vi "audio-stim2.vi"(11 "Stimulus List":dbl[][](array[numeric])) -> (3 "Playing":bool caption="Playing stimulus")   [LabVIEW 2009]
uses:
  <vilib>/DAQmx/create/channels.llb/DAQmx Create Channel (DO-Digital Output).vi
  <vilib>/DAQmx/write.llb/DAQmx Write (Digital U16 1Chan 1Samp).vi
  <vilib>/DAQmx/create/channels.llb/DAQmx Create Channel (AO-Voltage-Basic).vi
  <vilib>/DAQmx/write.llb/DAQmx Write (Analog Wfm 1Chan NSamp).vi
  <vilib>/DAQmx/configure/timing.llb/DAQmx Timing (Use Waveform).vi
panel:
  in  "Total Trials":i32 min=1 step=1
  out "Total Played":i32 caption="Total Played or Cued"
  in  "Save Stimulus List":bool
  in  "Load Stimulus List":bool
  out "Stimulus List Path":path
  out "Log File Path":path
  in  "Play Interval Jitter (s)":dbl
  in  "Play Interval (s)":dbl
  out "error out":errorcluster
  in  "DO Ports":tag caption="DO Ports\n(\"browse\" and select two 8 bit ports)"
  in  "Sound AO Channel":tag
  out "Curr Param":dbl[](array[numeric]) caption="Current (or Cued) Trial Parameters"
  in  "Sampling Rate":dbl
  in  "stop":bool
  in  "Play":bool
  out "Current (or Cued) Waveform":waveform(dbl)(graph)
  out "Waiting":bool
  # "Stim#, Stim Type, Duration, Amplitude, Param 1, Param 2, Param 3, Param 4"
  # "Stim Type 1 DC (no parameters, just amplitude)"
  # "Stim Type 3 Pure Tone (param1 = frequency)"
  # "Stim Type 4 FM Sweep (param1 = start frequency, param2 = end frequency)"
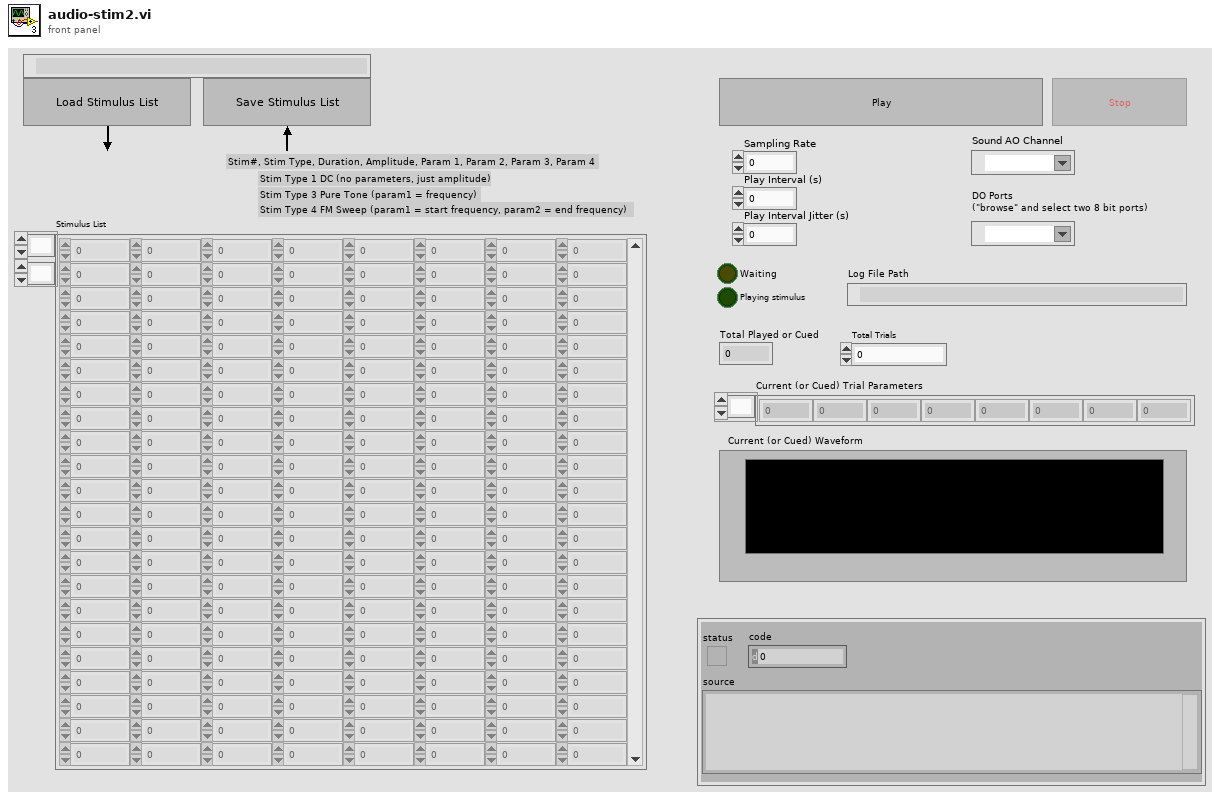
[diagram p1: front panel]
types:
  T1 = enum8{"Enabled", "Disabled", "Disabled and Grayed Out"}
  T2 = cluster{"Sampling Rate":dbl, "Value 3":dbl, dbl, "Value 2":dbl}
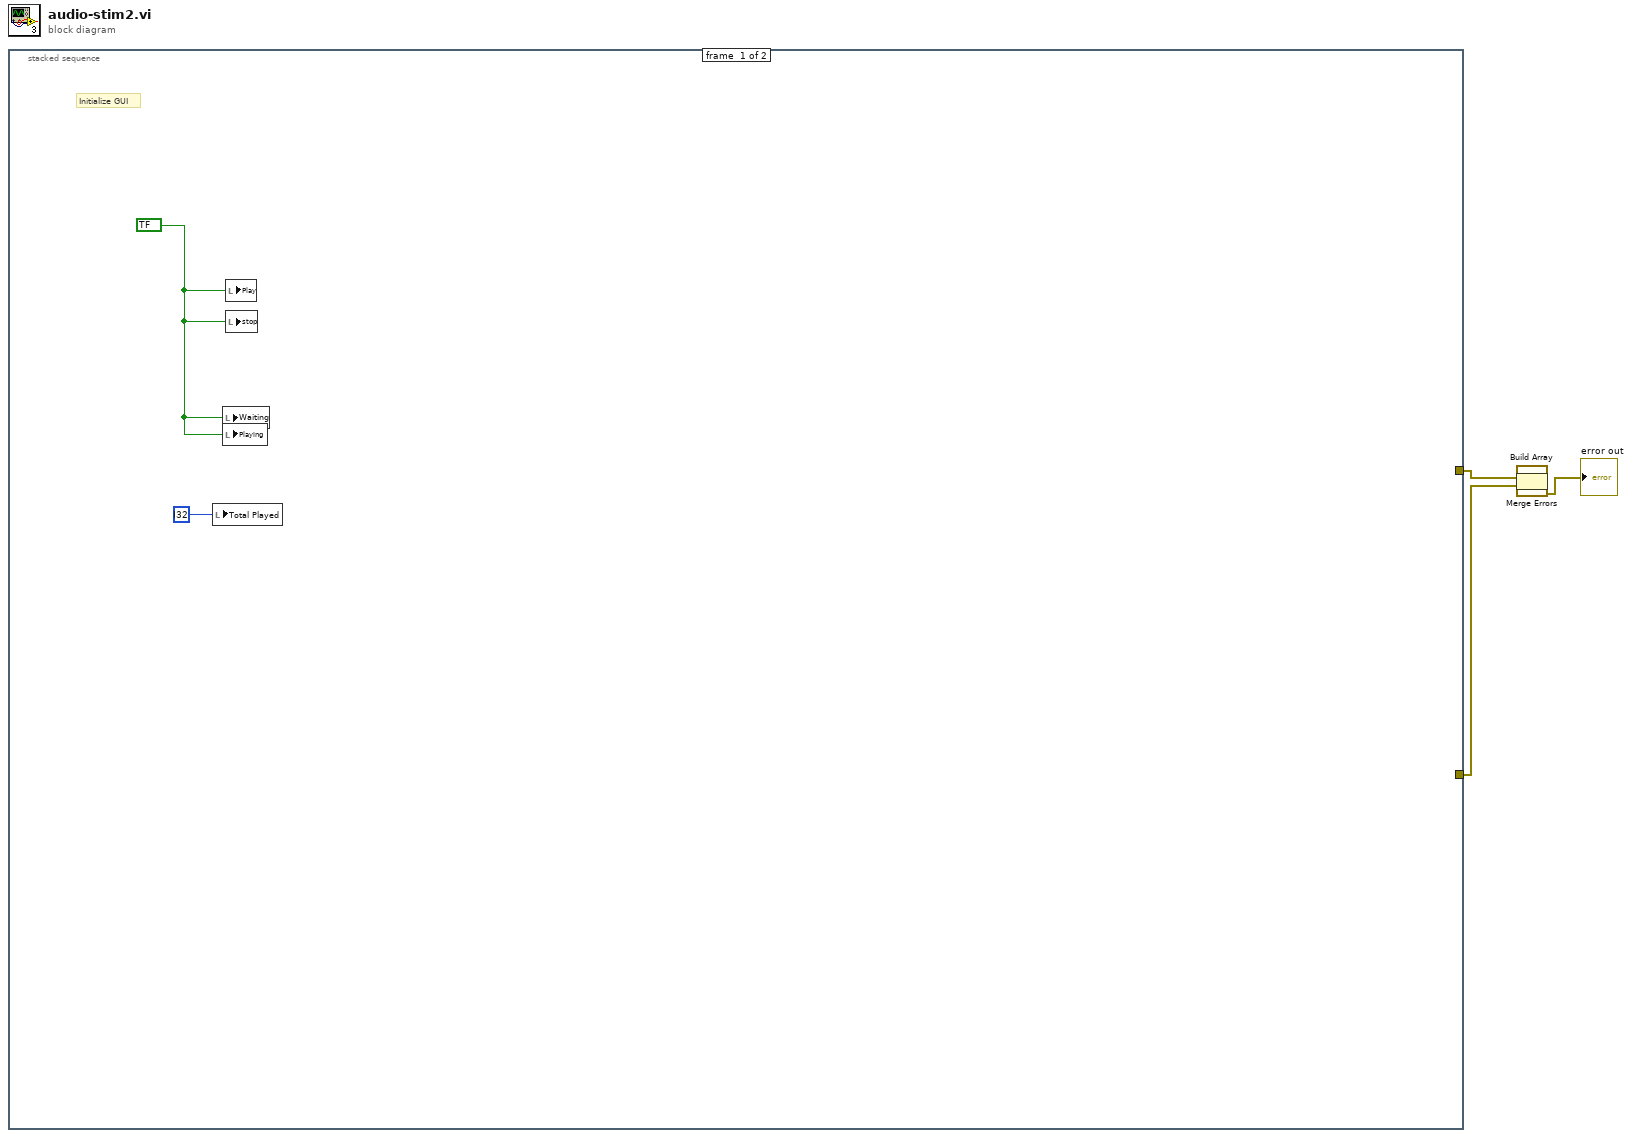
[diagram p0: block diagram]
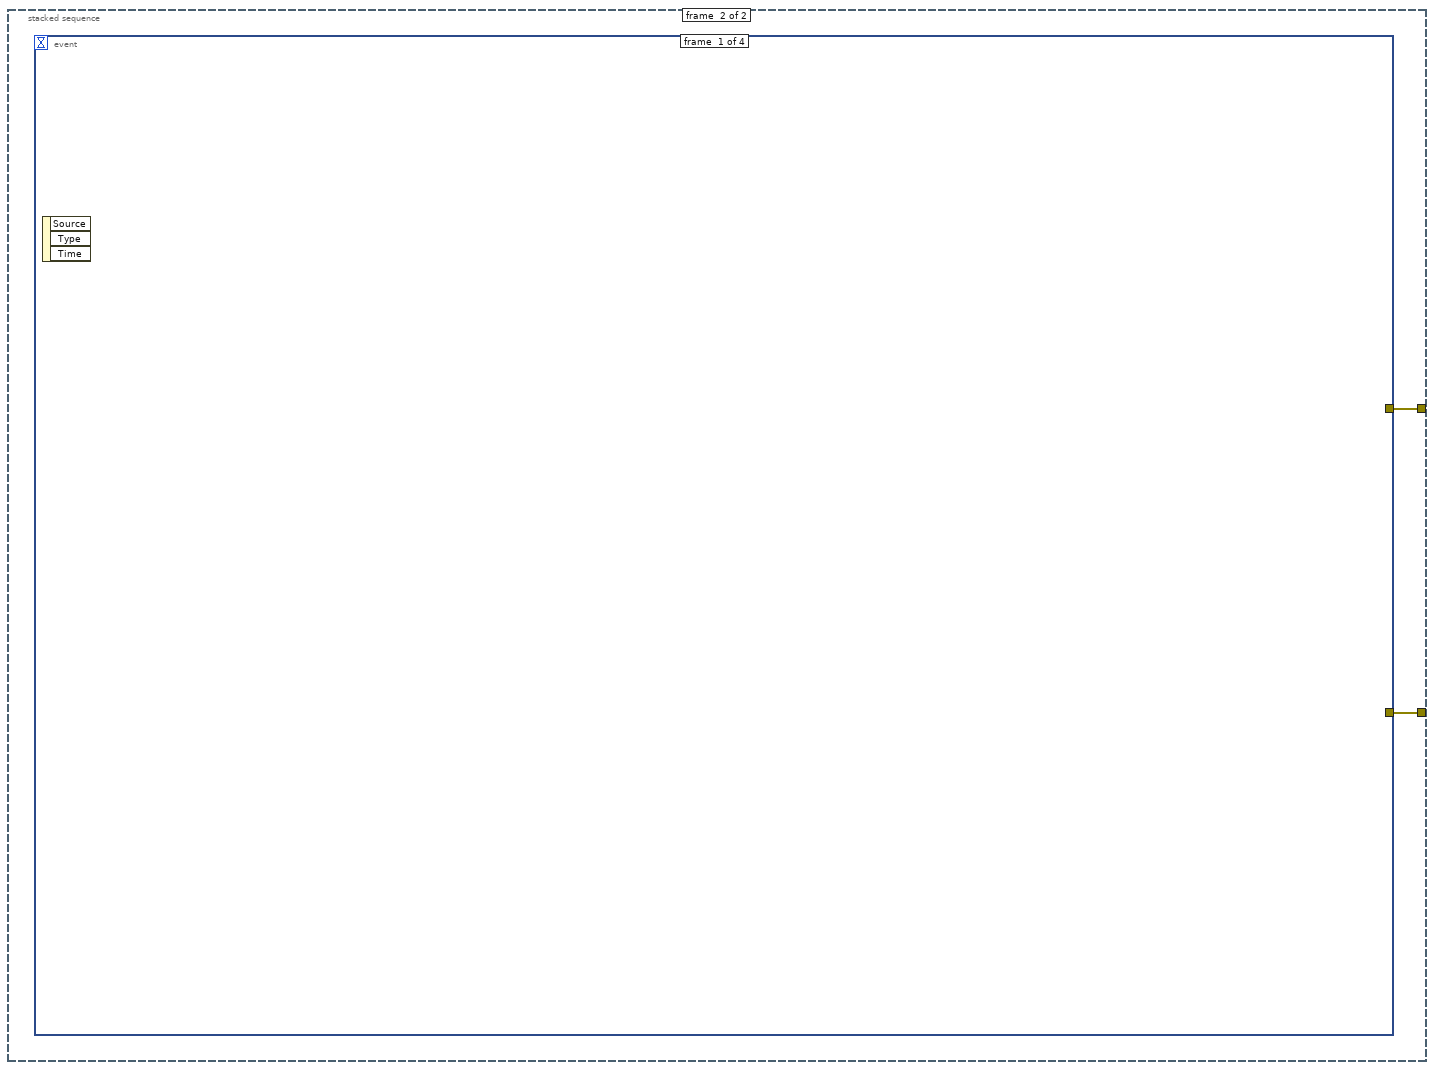
[diagram p2: hidden frame]
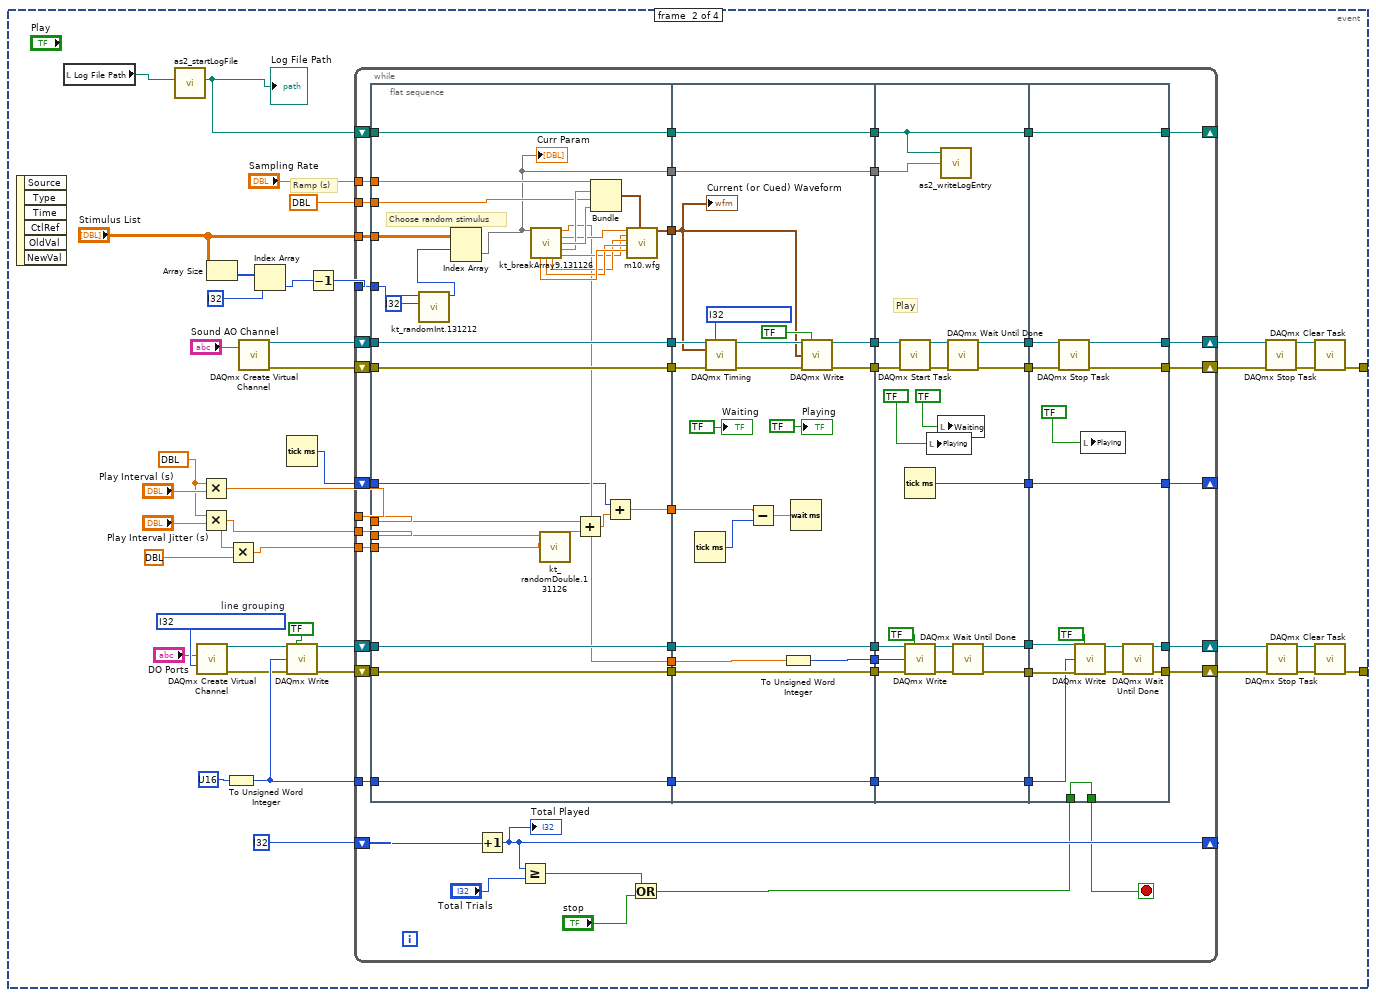
[diagram p3: hidden frame]
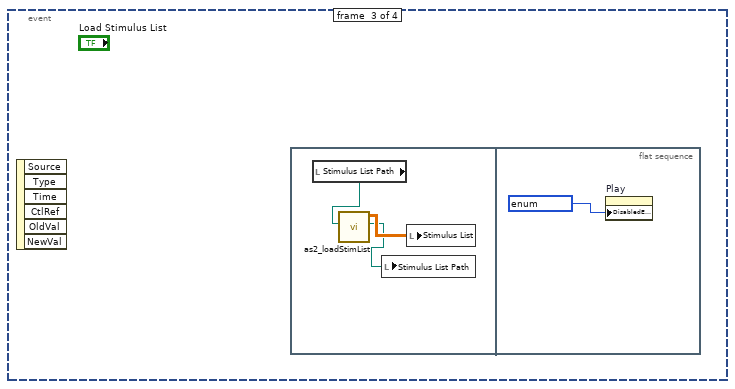
[diagram p4: hidden frame]
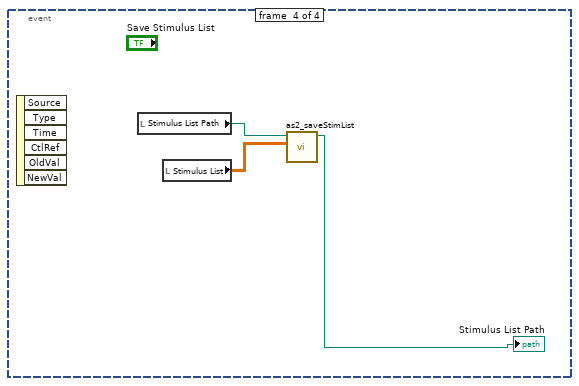
[diagram p5: hidden frame]
diagram:
  n1 = stacked-sequence {
    tunnel: [_ w8] -> w4
    tunnel: [_ w7] -> w3
    frame #0 {
      w6 = bool ? ("Play")
      # "Initialize GUI"
      n2 = local write "Total Played"(i32 ? ("Total Played")) -> ()
      n3 = local write "Waiting"(w6) -> ()
      n4 = local write "Playing"(w6) -> ()
      n5 = local write "Play"(w6) -> ()
      n6 = local write "stop"(w6) -> ()
    }
    frame #1 {
      n7 = event shown="[1] \"Play\": Value Change" {
        selector: _ -> [_ _ _ _]
        dyn-events: _ -> [_ _ _ _]
        timeout: _ -> [_ _ _ _]
        tunnel: [_ w25 _ _] -> w8
        tunnel: [_ w24 _ _] -> w7
        event #0 {
          n8 = event-data() -> ()  [unwired: 1 in, 3 out]
        }
        event #1 {
          w18 = dbl ? ("y")
          w45 = i32 ? items=["one channel for each line", "one channel for all lines"]  # line grouping
          # "Ramp (s)"
          n9 = event-data() -> ()  [unwired: 1 in, 6 out]
          n10 = local read "Log File Path"() -> (w13:path)
          n11 = call "as2_startLogFile.vi"("Path In"=w13) -> ("Path"=w12:path)  [unwired: 5 in, 1 out]
          "Log File Path" <- w12
          n12 = call-poly <vilib>:"DAQmx Create Virtual Channel.vi"("lines"="DO Ports", "line grouping"=w45) -> ("task out"=w23:refnum<k21>, "error out"=w22:errorcluster)  [unwired: 12 in]
          n13 = Multiply(x=w18, y="Play Interval (s)") -> (x*y=w17:dbl)
          n14 = Multiply(x=w18, y="Play Interval Jitter (s)") -> (x*y=w15:dbl)
          n15 = Array Size(array="Stimulus List") -> (size(s)=w43:i32[])
          n16 = To Unsigned Word Integer(number=u16 ? ("data")) -> (unsigned 16bit integer=w28:u16)
          n17 = Multiply(x=w15, y=dbl ?) -> (x*y=w16:dbl)
          n18 = call-poly <vilib>:"DAQmx Create Virtual Channel.vi"("physical channels"="Sound AO Channel") -> ("task out"=w27:refnum<k21>, "error out"=w26:errorcluster)  [unwired: 13 in]
          n19 = Index Array(array=w43, index=i32 ?) -> (element=w11:i32)
          n20 = Tick Count (ms)() -> (millisecond timer value=w14:u32)
          n21 = call-poly <vilib>:"DAQmx Write.vi"("task/channels in"=w23, "auto start"=bool ?, "data"=w28, "error in"=w22) -> ("task out"=w32:refnum<k21>, "error out"=w31:errorcluster)  [unwired: 9 in, 1 out]
          n22 = Decrement(x=w11) -> (x-1=w10:i32)
          n23 = while {
            tunnel: "Stimulus List" -> [w73]
            tunnel: "Sampling Rate" -> [w72]
            tunnel: dbl ? -> [w71]
            shift-right: [w98] -> w37
            shift-left: w27 -> [w96]
            shift-right: [w97] -> w36
            shift-left: w26 -> [w95]
            shift-right: [w87] -> w41
            shift-left: w32 -> [w94]
            shift-right: [w86] -> w40
            shift-left: w31 -> [w81]
            shift-right: [w52] -> _
            shift-left: i32 ? ("data") -> [w53]
            tunnel: w28 -> [w84]
            shift-right: [w68] -> _
            shift-left: w14 -> [w67]
            tunnel: w17 -> [w63]
            tunnel: w16 -> [w64]
            tunnel: w15 -> [w65]
            shift-right: [w56] -> _
            shift-left: w12 -> [w62]
            tunnel: w10 -> [w55]
            stop <- w50 stop-if-true
            n24 = flat-sequence {
              tunnel: [w130] -> w79
              tunnel: [w129] -> w78
              tunnel: [w128] -> w77
              tunnel: [w127] -> w76
              tunnel: [w126] -> w75
              tunnel: [w118] -> w74
              tunnel: [w115] -> w70
              tunnel: [w112] -> w66
              tunnel: [w106] -> w61
              tunnel: [w105] -> w60
              tunnel: w55 -> [w104]
              tunnel: w62 -> [w106]
              tunnel: w63 -> [w107]
              tunnel: w64 -> [w110]
              tunnel: w65 -> [w111]
              tunnel: w67 -> [w113]
              tunnel: w71 -> [w116]
              tunnel: w72 -> [w117]
              tunnel: w73 -> [w102]
              tunnel: w81 -> [w126]
              tunnel: w84 -> [w127]
              tunnel: w94 -> [w128]
              tunnel: w95 -> [w129]
              tunnel: w96 -> [w130]
              tunnel: [w141] -> w100
              tunnel: [w140] -> w99
              tunnel: [w150] -> w93
              tunnel: [w149] -> w88
              tunnel: [w148] -> w85
              tunnel: [w138] -> w80
              tunnel: w79 -> [w147]
              tunnel: w78 -> [w146]
              tunnel: w77 -> [w150]
              tunnel: w76 -> [w148]
              tunnel: w75 -> [w138]
              tunnel: w74 -> [w137]
              tunnel: w70 -> [w136]
              tunnel: w66 -> [w133]
              tunnel: w61 -> [w131]
              tunnel: w60 -> [w132]
              tunnel: [w132] -> w59
              tunnel: [w131] -> w58
              tunnel: w100 -> [w161]
              tunnel: w99 -> [w160]
              tunnel: w93 -> [w169]
              tunnel: [w163] -> w92
              tunnel: [w162] -> w91
              tunnel: [w166] -> w90
              tunnel: [w165] -> w89
              tunnel: w88 -> [w170]
              tunnel: w85 -> [w164]
              tunnel: [w164] -> w83
              tunnel: w80 -> [w155]
              tunnel: [w154] -> w69
              tunnel: w59 -> [w153]
              tunnel: w58 -> [w152]
              tunnel: [w152] -> w57
              tunnel: [w175] -> w97
              tunnel: [w176] -> w98
              tunnel: w92 -> [w178]
              tunnel: w91 -> [w177]
              tunnel: w90 -> [w186]
              tunnel: w89 -> [w185]
              tunnel: [w181] -> w87
              tunnel: [w180] -> w86
              tunnel: w83 -> [w179]
              tunnel: w69 -> [w174]
              tunnel: [w174] -> w68
              tunnel: w57 -> [w173]
              tunnel: [w173] -> w56
              tunnel: w51 -> [w172]
              tunnel: [w172] -> w50
              frame #0 {
                # "Choose random stimulus"
                n25 = call "kt_randomInt.131212.vi"("Min"=i32 ?, "Max"=w104) -> ("Random"=w101:i32)  [unwired: 9 in]
                n26 = Index Array(array=w102, index (row)=w101) -> (element=w105:dbl[])  [unwired: 1 in]
                "Curr Param" <- w105
                n27 = call "kt_breakArray9.131126.vi"("Current (or Cued Trial Parameters)"=w105) -> ("Value 0"=w115:dbl, "Value 1"=w119:dbl, "Value 2"=w121:dbl, "Value 3"=w120:dbl, "Value 7"=w125:dbl, "Value 6"=w124:dbl, "Value 5"=w123:dbl, "Value 4"=w122:dbl)  [unwired: 6 in, 1 out]
                n28 = call "kt_randomDouble.131126.vi"("Min"=w110, "Max"=w111) -> ("Random"=w108:dbl)  [unwired: 9 in]
                n29 = Add(x=w107, y=w108) -> (x+y=w109:dbl)
                n30 = Bundle("Sampling Rate"=w117, "Value 3"=w120, w116, "Value 2"=w121) -> (w114:T2)  [unwired: 1 in]
                n31 = Add(x=w113, y=w109) -> (x+y=w112:dbl)
                n32 = call "m10.wfg.vi"("Stimulus Type"=w119, "Param 0"=w122, "Param 1"=w123, "Param 2"=w124, "Param 3"=w125, "Waveform Properties"=w114) -> ("Waveform Out"=w118:waveform(dbl))  [unwired: 12 in, 1 out]
              }
              frame #1 {
                w145 = i32 ? items=["Finite Samples", "Continuous Samples", "Hardware Timed Single Point"] ("sample mode")
                n33 = Tick Count (ms)() -> (millisecond timer value=w134:u32)
                n34 = call-poly <vilib>:"DAQmx Timing.vi"("task/channels in"=w147, "sample mode"=w145, "waveform"=w137, "error in"=w146) -> ("task out"=w144:refnum<k21>, "error out"=w143:errorcluster)  [unwired: 10 in]
                n35 = Subtract(x=w133, y=w134) -> (x-y=w135:dbl)
                n36 = To Unsigned Word Integer(number=w136) -> (unsigned 16bit integer=w149:u16)
                n37 = Wait (ms)(milliseconds to wait=w135) -> ()  [unwired: 1 out]
                n38 = call-poly <vilib>:"DAQmx Write.vi"("task/channels in"=w144, "auto start"=bool ?, "data"=w137, "error in"=w143) -> ("task out"=w141:refnum<k21>, "error out"=w140:errorcluster)  [unwired: 9 in, 1 out]
                "Waiting" <- bool ? ("Playing Stimulus")
                "Playing" <- bool ? ("Playing Stimulus")
                "Current (or Cued) Waveform" <- w137
              }
              frame #2 {
                # "Play"
                n39 = call <vilib>:"DAQmx Start Task.vi"("task/channels in"=w161, "error in"=w160) -> ("task out"=w159:refnum<k21>, "error out"=w158:errorcluster)  [unwired: 12 in]
                n40 = Tick Count (ms)() -> (millisecond timer value=w154:u32)
                n41 = call-poly <vilib>:"DAQmx Write.vi"("task/channels in"=w169, "auto start"=bool ?, "data"=w170, "error in"=w155) -> ("task out"=w168:refnum<k21>, "error out"=w167:errorcluster)  [unwired: 9 in, 1 out]
                n42 = local write "Playing"(bool ? ("Playing Stimulus")) -> ()
                n43 = local write "Waiting"(bool ? ("Playing Stimulus")) -> ()
                n44 = call "as2_writeLogEntry.vi"("Path In"=w152, "Curr Param"=w153) -> ()  [unwired: 4 in, 1 out]
                n45 = call <vilib>:"DAQmx Wait Until Done.vi"("task/channels in"=w159, "error in"=w158) -> ("task out"=w163:refnum<k21>, "error out"=w162:errorcluster)  [unwired: 12 in]
                n46 = call <vilib>:"DAQmx Wait Until Done.vi"("task/channels in"=w168, "error in"=w167) -> ("task out"=w166:refnum<k21>, "error out"=w165:errorcluster)  [unwired: 12 in]
              }
              frame #3 {
                n47 = call <vilib>:"DAQmx Stop Task.vi"("task/channels in"=w178, "error in"=w177) -> ("task out"=w176:refnum<k21>, "error out"=w175:errorcluster)  [unwired: 12 in]
                n48 = call-poly <vilib>:"DAQmx Write.vi"("task/channels in"=w186, "auto start"=bool ?, "data"=w179, "error in"=w185) -> ("task out"=w183:refnum<k21>, "error out"=w182:errorcluster)  [unwired: 9 in, 1 out]
                n49 = local write "Playing"(bool ? ("Playing Stimulus")) -> ()
                n50 = call <vilib>:"DAQmx Wait Until Done.vi"("task/channels in"=w183, "error in"=w182) -> ("task out"=w181:refnum<k21>, "error out"=w180:errorcluster)  [unwired: 12 in]
              }
            }
            n51 = Increment(x=w53) -> (x+1=w52:i32)
            "Total Played" <- w52
            n52 = Greater Or Equal?(x=w52, y="Total Trials") -> (x >= y?=w82:bool)
            n53 = Or(x=w82, y="stop") -> (x .or. y?=w51:bool)
          }
          n54 = call <vilib>:"DAQmx Stop Task.vi"("task/channels in"=w37, "error in"=w36) -> ("task out"=w35:refnum<k21>, "error out"=w34:errorcluster)  [unwired: 12 in]
          n55 = call <vilib>:"DAQmx Stop Task.vi"("task/channels in"=w41, "error in"=w40) -> ("task out"=w39:refnum<k21>, "error out"=w38:errorcluster)  [unwired: 12 in]
          n56 = call <vilib>:"DAQmx Clear Task.vi"("task in"=w35, "error in"=w34) -> ("error out"=w25:errorcluster)  [unwired: 13 in]
          n57 = call <vilib>:"DAQmx Clear Task.vi"("task in"=w39, "error in"=w38) -> ("error out"=w24:errorcluster)  [unwired: 13 in]
        }
        event #2 {
          n58 = event-data() -> ()  [unwired: 1 in, 6 out]
          n59 = flat-sequence {
            frame #0 {
              n60 = local read "Stimulus List Path"() -> (w190:path)
              n61 = call "as2_loadStimList.vi"("Path In"=w190) -> ("Path"=w188:path, "Stimulus List"=w189:dbl[][])  [unwired: 4 in, 1 out]
              n62 = local write "Stimulus List Path"(w188) -> ()
              n63 = local write "Stimulus List"(w189) -> ()
            }
            frame #1 {
              n64 = property on="Play" class="Bool (strict)"("DisabledEnum"=T1 ? ("Disabled")) -> ()  [unwired: 2 in, 2 out]
            }
          }
        }
        event #3 {
          n65 = event-data() -> ()  [unwired: 1 in, 6 out]
          n66 = local read "Stimulus List Path"() -> (w194:path)
          n67 = local read "Stimulus List"() -> (w193:dbl[][])
          n68 = call "as2_saveStimList.vi"("Stimulus List"=w193, "Path In"=w194) -> ("Path"=→"Stimulus List Path":path)  [unwired: 4 in, 1 out]
        }
      }
    }
  }
  n69 = Build Array(w4, w3) -> (w1:errorcluster[])
  n70 = call <vilib>:"Merge Errors.vi"("error array in"=w1) -> ("error out"=→"error out":errorcluster)  [unwired: 6 in]
